vi "Log Errors and Warnings.vi"(8 "error in (no error)":errorcluster, 10 "Location":string, 11 "Process In":refnum<class "Process.lvclass">) -> (0 "error out":errorcluster, 3 "Process Out":refnum<class "Process.lvclass">)   [LabVIEW 2020, in "Process.lvclass"]
doc: "Log errors and warnings to all configured log handlers."
uses:
  Process.lvclass
  C:/git/astemes-triarc-framework/source/Framework/Logging/Logging.lvclass
  Logging/Logging.lvclass
  Process.lvclass/Process.ctl
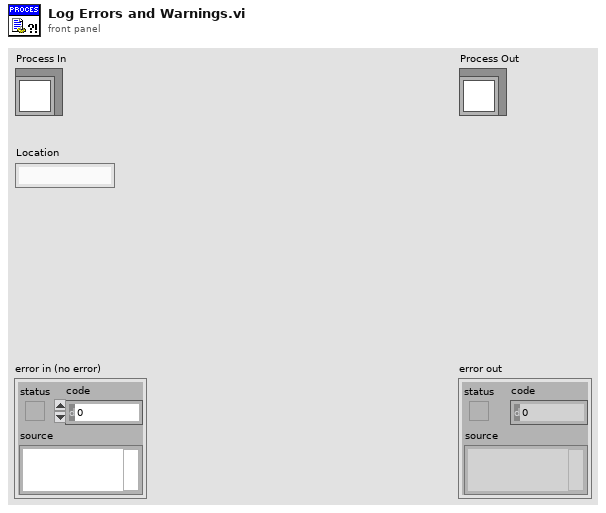
[diagram p1: front panel]
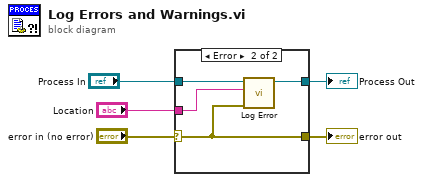
[diagram p0: block diagram]
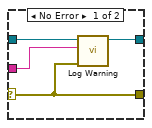
[diagram p2: hidden frame]
diagram:
  n1 = case shown="Error" "error in (no error)" {
    selector: "error in (no error)" -> [w6 w10]
    tunnel: [w6 w10] -> w4
    tunnel: [w9 w13] -> w2
    tunnel: "Process In" -> [w8 w12]
    tunnel: "Location" -> [w7 w11]
    frame No Error {
      n2 = call "Log Warning.vi"("error in (no error)"=w6, "Message"=w7, "Logging In"=w8) -> ("Logging Out"=w9:refnum<class "Process.lvclass">)  [unwired: 7 in, 1 out]
    }
    frame Error {
      n3 = call "Log Error.vi"("error in (no error)"=w10, "Message"=w11, "Logging In"=w12) -> ("Logging Out"=w13:refnum<class "Process.lvclass">)  [unwired: 7 in, 1 out]
    }
  }
  "error out" <- w4
  "Process Out" <- w2
